vi "exercise3_arraysine.vi"() -> ()   [LabVIEW 2018]
panel:
  out "Waveform Array 2":dbl[](graph)
  out "Waveform Array 3":waveform(dbl)(graph)
  out "Waveform Array 1":dbl[](graph)
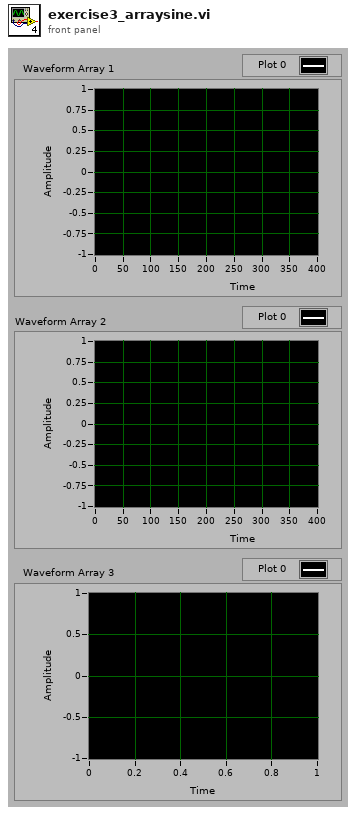
[diagram p1: front panel]
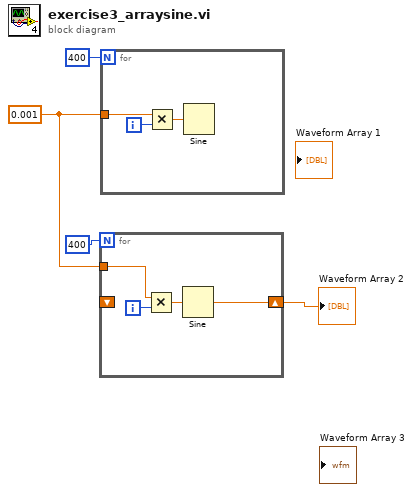
[diagram p0: block diagram]
diagram:
  w1 = 0.001 ("x 2")
  n1 = for {
    N: 400 -> [_]
    shift-right: [w6] -> w2
    shift-left: _ -> [_]
    tunnel: w1 -> [w5]
    i -> [w7]
    n2 = Multiply(x=w5, y=w7) -> (x*y=w8:dbl)
    n3 = Sine(x=w8) -> (sin(x)=w6:dbl)
  }
  "Waveform Array 2" <- w2
  n4 = for {
    N: 400 -> [_]
    tunnel: w1 -> [w9]
    i -> [w10]
    n5 = Multiply(x=w9, y=w10) -> (x*y=w11:dbl)
    n6 = Sine(x=w11) -> ()  [unwired: 1 out]
  }
